vi "LVClass_Camera get ALLParameter.vi"(0 "Camera in":refnum<class "Camera.lvclass">, 11 "error in (no error)":errorcluster) -> (4 "Camera out":refnum<class "Camera.lvclass">, 6 "ListOfSettableAndGettableValue":T1[](array[typedef]), 8 "nb_image":u32, 10 "BG Image OUT":refnum<class "Image.lvclass">, 15 "error out":errorcluster)   [LabVIEW 2020, in "Camera.lvclass"]
doc: "Get camera parameters which are gettable and settable parameter \n\n<B>CameraIn</B> : Camera object.\n<B>CameraOut</B> : Camera object.\n<B>BG Image OUIT</B> : Defined background image object if it is allready defined throught camera object method \"LVClass_Camera set background.vi\".\nThis image object is a reference : DO NOT DELETE THIS OBJECT BY YOURSELF\n<B>nb_image</B> : number of summed of images\n<B>ListOfSettableAndGettableValue</B> : Array of the parameter with readen value from camera object."
uses:
  Camera.lvclass
  CameraParametersSetup.ctl
  CameraParameters_Type.ctl
  Image.lvclass
  Camera.lvclass/Camera.ctl
  LVClass_Camera Read acquisition state.vi
  LVClass_Camera Read all camera parameters.vi
  LVClass_Image read Image Compat ptr.vi
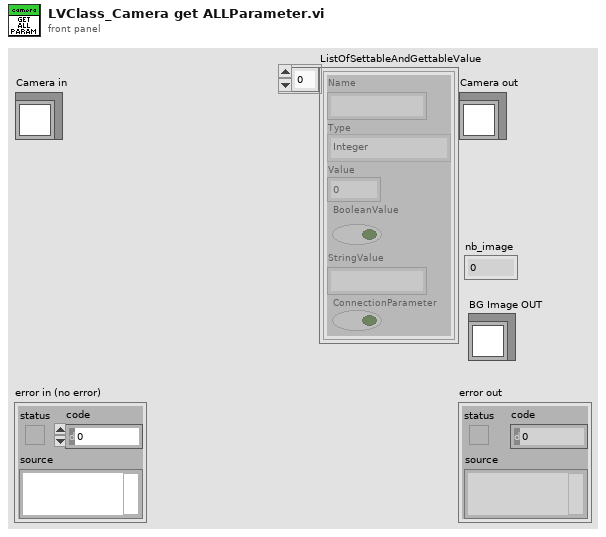
[diagram p1: front panel]
types:
  T1 = typedef "CameraParametersSetup.ctl" = cluster{"Name":string, "Type":T2, "Value":dbl, "BooleanValue":bool, "StringValue":string, "ConnectionParameter":bool}
  T2 = typedef "CameraParameters_Type.ctl" = enum16{"Integer", "Real", "String", "Boolean"}
  T3 = typedef "CameraAcquisitionState.ctl" = enum16{"Stop", "Live"}
  T4 = typedef "ParameterID.ctl" = cluster{"Name":string, "ConnectionParameter?":bool, "Type":T2, "Authorization":T5, "OnFlyAuthorization":T6, "StringValue":string, "Value":dbl, "Min":dbl, "Max":dbl, "BooleanValue":bool, "StringParameterList":string[]}
  T5 = typedef "CameraParameters_Authorization.ctl" = enum16{"Disable", "Gettable", "Settable - Gettable"}
  T6 = typedef "CameraParameters_OnFlyAuthorization.ctl" = enum16{"None", "Gettable", "Settable", "Settable - Gettable"}
  T7 = typedef "ClassID.ctl" = i64
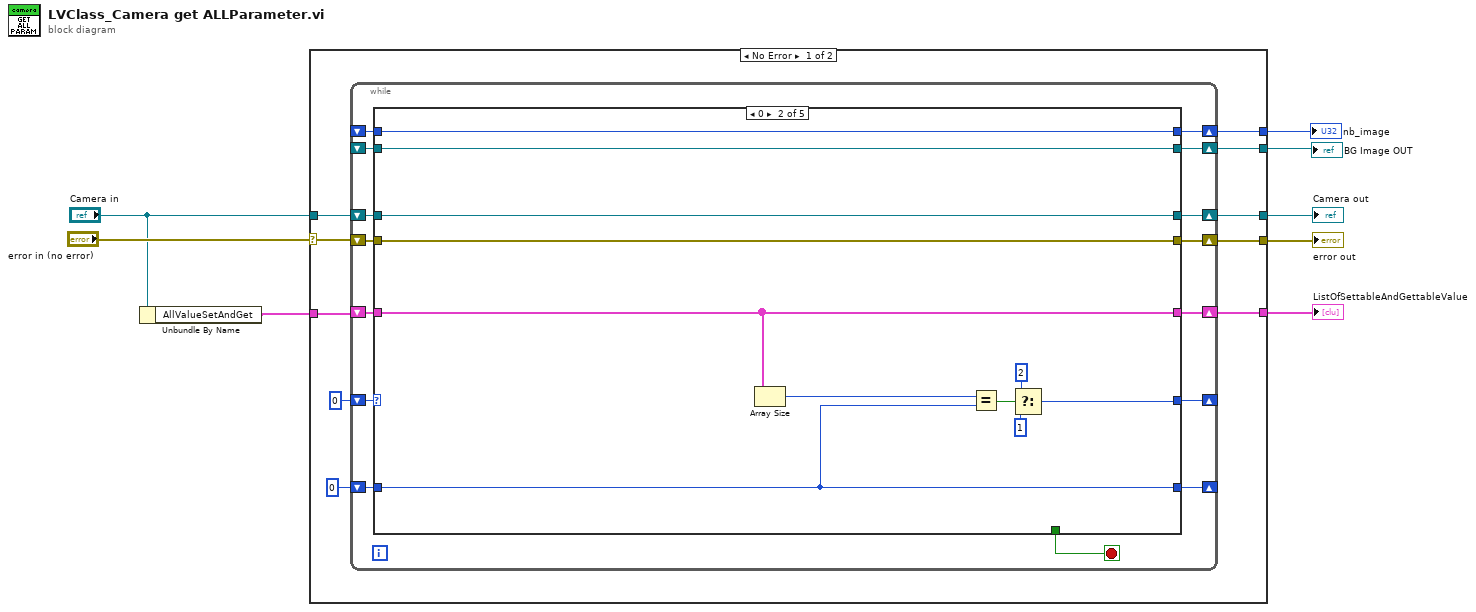
[diagram p0: block diagram]
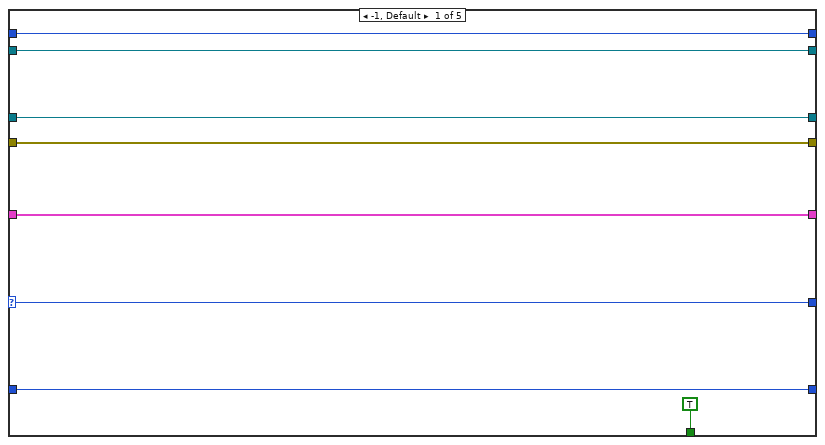
[diagram p2: hidden frame]
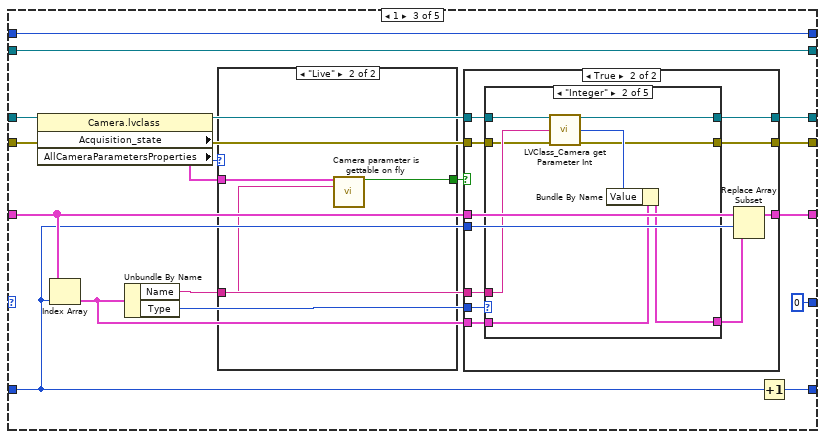
[diagram p3: hidden frame]
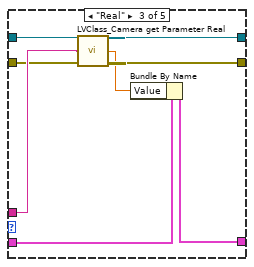
[diagram p6: hidden frame]
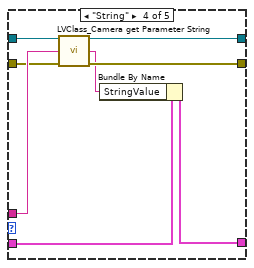
[diagram p7: hidden frame]
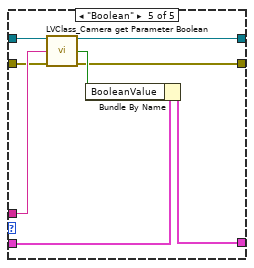
[diagram p8: hidden frame]
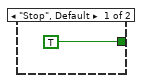
[diagram p9: hidden frame]
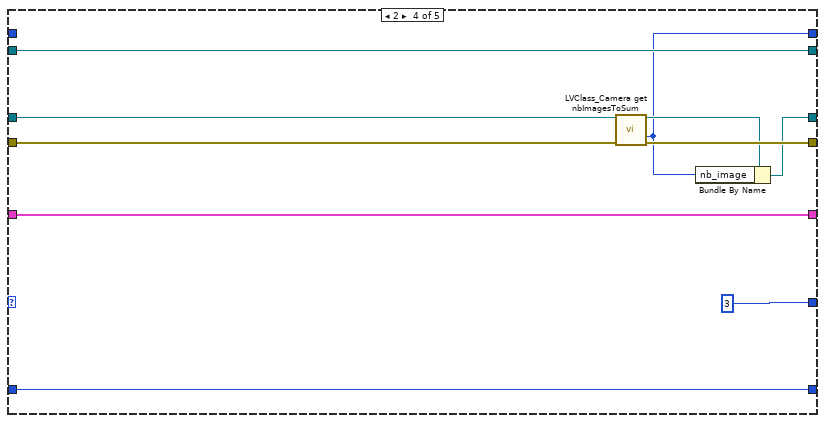
[diagram p10: hidden frame]
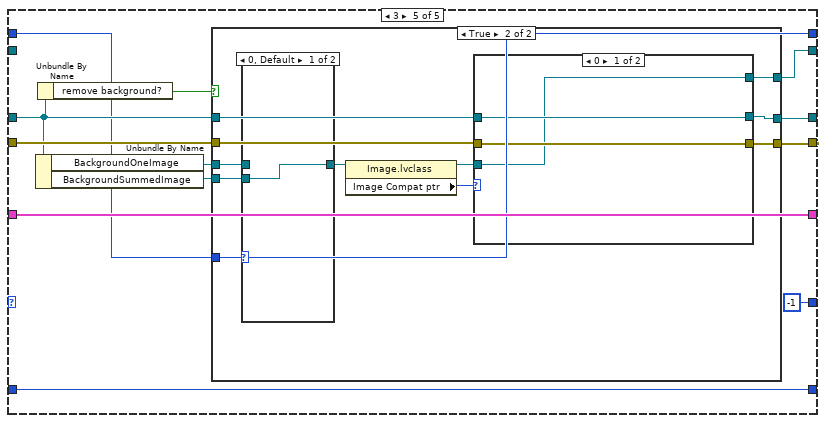
[diagram p11: hidden frame]
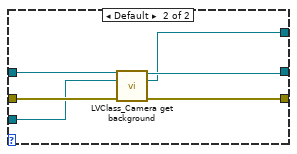
[diagram p14: hidden frame]
diagram:
  n1 = Unbundle By Name("Camera in") -> ("AllValueSetAndGet"=w1:T1[])
  n2 = case shown="No Error" "error in (no error)" {
    selector: "error in (no error)" -> [w14 w173]
    tunnel: [w15 w173] -> w7
    tunnel: [w16 w172] -> w6
    tunnel: "Camera in" -> [w18 w172]
    tunnel: [w13 _] -> w5
    tunnel: [w12 _] -> w4
    tunnel: [w11 _] -> w3
    tunnel: w1 -> [w9 _]
    frame No Error {
      n3 = while {
        shift-right: [w32] -> _
        shift-left: 0 -> [w31]
        shift-right: [w29] -> w15
        shift-left: w14 -> [w28]
        shift-right: [w30] -> w16
        shift-left: w18 -> [w33]
        shift-right: [w25] -> w13
        shift-left: _ -> [w26]
        shift-right: [w24] -> w12
        shift-left: w9 -> [w23]
        shift-right: [w22] -> w11
        shift-left: _ -> [w21]
        shift-right: [w19] -> _
        shift-left: 0 -> [w20]
        stop <- w27 stop-if-true
        n4 = case shown="0" w31 {
          selector: w31 -> [w34 _ _ _ _]
          tunnel: w33 -> [w40 w52 w60 w133 w140]
          tunnel: w28 -> [w39 w51 w58 w132 w146]
          tunnel: [w34 w43 0 3 -1] -> w32
          tunnel: [w40 w52 w70 w127 w145] -> w30
          tunnel: [w39 w51 w69 w131 w144] -> w29
          tunnel: [TRUE _ _ _ _] -> w27
          tunnel: w26 -> [w38 w50 w68 w130 _]
          tunnel: [w38 w50 w68 w130 w143] -> w25
          tunnel: [w36 w48 w62 w129 w142] -> w24
          tunnel: w23 -> [w36 w48 w64 w129 w142]
          tunnel: [w37 w49 w67 w126 w137] -> w22
          tunnel: w21 -> [w37 w49 w67 _ w137]
          tunnel: w20 -> [w35 w46 w63 w125 w135]
          tunnel: [w35 w46 w66 w125 w135] -> w19
          frame -1, Default {
          }
          frame 0 {
            n5 = Array Size(array=w48) -> (size(s)=w47:i32)
            n6 = Equal?(x=w47, y=w46) -> (x = y?=w45:bool)
            n7 = Select(t=2, s=w45, f=1) -> (s? t:f=w43:i32)
          }
          frame 1 {
            n8 = property class="Camera.lvclass"(reference=w60, error in=w58) -> (reference out=w59:refnum<class "Camera.lvclass">, error out=w57:errorcluster, "Acquisition_state"=w56:T3, "AllCameraParametersProperties"=w55:T4[])
            n9 = Index Array(array=w64, index=w63) -> (element=w65:T1)
            n10 = Unbundle By Name(w65) -> ("Name"=w53:string, "Type"=w61:T2)
            n11 = case shown="\"Live\"" w56 {
              tunnel: w55 -> [_ w123]
              tunnel: [TRUE w124] -> w54
              tunnel: w53 -> [_ w122]
              frame "Stop", Default {
              }
              frame "Live" {
                n12 = call "Camera parameter is gettable on fly.vi"("AllCameraParameters"=w123, "Name"=w122) -> ("Gettable?"=w124:bool)  [unwired: 13 in]
              }
            }
            n13 = case shown="True" w54 {
              tunnel: [w74 w85] -> w70
              tunnel: [w73 w84] -> w69
              tunnel: w65 -> [_ w83]
              tunnel: w64 -> [w72 w82]
              tunnel: w63 -> [_ w81]
              tunnel: [w72 w80] -> w62
              tunnel: w61 -> [_ w79]
              tunnel: w53 -> [_ w78]
              tunnel: w59 -> [w74 w77]
              tunnel: w57 -> [w73 w76]
              frame False {
              }
              frame True {
                n14 = case shown="\"Integer\"" w79 {
                  tunnel: w83 -> [w86 w96 w97 w105 w114]
                  tunnel: [w86 w95 w98 w112 w113] -> w75
                  tunnel: w78 -> [_ w94 w103 w109 w119]
                  tunnel: w77 -> [w88 w93 w104 w111 w120]
                  tunnel: [w88 w92 w100 w110 w117] -> w85
                  tunnel: [w87 w90 w101 w107 w115] -> w84
                  tunnel: w76 -> [w87 w89 w102 w108 w118]
                  frame Default {
                  }
                  frame "Integer" {
                    n15 = call "LVClass_Camera get Parameter Int.vi"("Camera in"=w93, "parameter_name"=w94, "error in (no error)"=w89) -> ("Camera out"=w92:refnum<class "Camera.lvclass">, "value"=w91:i32, "error out"=w90:errorcluster)  [unwired: 10 in]
                    n16 = Bundle By Name(cluster=w96, "Value"=w91) -> (w95:T1)
                  }
                  frame "Real" {
                    n17 = call "LVClass_Camera get Parameter Real.vi"("Camera in"=w104, "parameter_name"=w103, "error in (no error)"=w102) -> ("Camera out"=w100:refnum<class "Camera.lvclass">, "value"=w99:dbl, "error out"=w101:errorcluster)  [unwired: 10 in]
                    n18 = Bundle By Name(cluster=w97, "Value"=w99) -> (w98:T1)
                  }
                  frame "String" {
                    n19 = call "LVClass_Camera get Parameter String.vi"("Camera in"=w111, "parameter_name"=w109, "error in (no error)"=w108) -> ("Camera out"=w110:refnum<class "Camera.lvclass">, "value"=w106:string, "error out"=w107:errorcluster)  [unwired: 10 in]
                    n20 = Bundle By Name(cluster=w105, "StringValue"=w106) -> (w112:T1)
                  }
                  frame "Boolean" {
                    n21 = call "LVClass_Camera get Parameter Boolean.vi"("Camera in"=w120, "parameter_name"=w119, "error in (no error)"=w118) -> ("Camera out"=w117:refnum<class "Camera.lvclass">, "value"=w116:bool, "error out"=w115:errorcluster)  [unwired: 10 in]
                    n22 = Bundle By Name(cluster=w114, "BooleanValue"=w116) -> (w113:T1)
                  }
                }
                n23 = Replace Array Subset(array=w82, new element=w75, index=w81) -> (w80:T1[])
              }
            }
            n24 = Increment(x=w63) -> (x+1=w66:i32)
          }
          frame 2 {
            n25 = call "LVClass_Camera get nbImagesToSum.vi"("Camera in"=w133, "error in (no error)"=w132) -> ("Camera out"=w128:refnum<class "Camera.lvclass">, "nb_image"=w126:u32, "error out"=w131:errorcluster)  [unwired: 11 in]
            n26 = Bundle By Name(cluster=w128, "nb_image"=w126) -> (w127:refnum<class "Camera.lvclass">)
          }
          frame 3 {
            n27 = Unbundle By Name(w140) -> ("BackgroundOneImage"=w141:refnum<class "Image.lvclass">, "BackgroundSummedImage"=w136:refnum<class "Image.lvclass">)
            n28 = Unbundle By Name(w140) -> ("remove background?"=w138:bool)
            n29 = case shown="True" w138 {
              tunnel: w146 -> [w147 w159]
              tunnel: [w148 w158] -> w145
              tunnel: [w147 w157] -> w144
              tunnel: [w149 w156] -> w143
              tunnel: w141 -> [w149 w152]
              tunnel: w140 -> [w148 w155]
              tunnel: w137 -> [_ w153]
              tunnel: w136 -> [_ w150]
              frame False {
              }
              frame True {
                n30 = case shown="0, Default" w153 {
                  tunnel: w152 -> [_ w162]
                  tunnel: [w161 w162] -> w151
                  tunnel: w150 -> [w161 _]
                  frame 0, Default {
                  }
                  frame 1 {
                  }
                }
                n31 = property class="Image.lvclass"(reference=w151) -> (reference out=w154:refnum<class "Image.lvclass">, "Image Compat ptr"=w160:T7)  [unwired: 1 in, 1 out]
                n32 = case shown="0" w160 {
                  tunnel: w155 -> [w164 w171]
                  tunnel: w159 -> [w165 w170]
                  tunnel: [w164 w169] -> w158
                  tunnel: [w165 w168] -> w157
                  tunnel: [w163 w167] -> w156
                  tunnel: w154 -> [w163 w166]
                  frame 0 {
                  }
                  frame Default {
                    n33 = call "LVClass_Camera get background.vi"("Camera in"=w171, "BG Image IN"=w166, "error in (no error)"=w170) -> ("Camera out"=w169:refnum<class "Camera.lvclass">, "BG Image OUT"=w167:refnum<class "Image.lvclass">, "error out"=w168:errorcluster)  [unwired: 10 in]
                  }
                }
              }
            }
          }
        }
      }
    }
    frame Error {
    }
  }
  "error out" <- w7
  "Camera out" <- w6
  "ListOfSettableAndGettableValue" <- w4
  "nb_image" <- w3
  "BG Image OUT" <- w5
